vi "register_data_from_termocuple.vi"(8 "error in (no error)":errorcluster, 11 "DAQ Voltage in":refnum<class "DAQ Voltage.lvclass">) -> (0 "error out":errorcluster, 3 "DAQ Voltage out":refnum<class "DAQ Voltage.lvclass">)   [LabVIEW 2025, in "DAQ Voltage.lvlib" / "DAQ Voltage.lvclass"]
uses:
  DAQ Voltage.lvclass
  DAQ Voltage.lvclass/DAQ Voltage.ctl
  <vilib>/numeric/Random Number (Range) DBL.vi
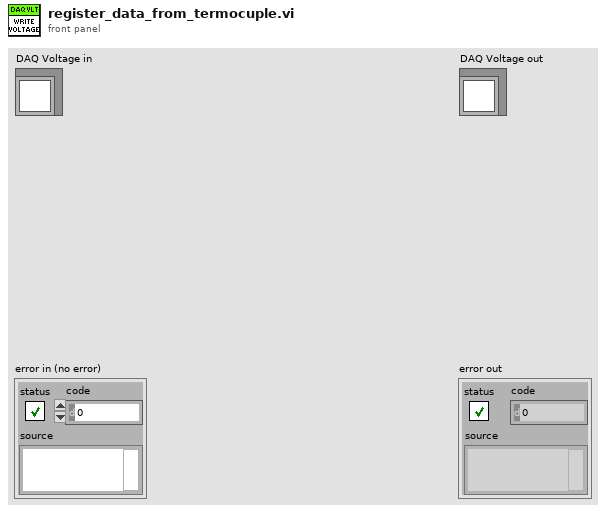
[diagram p1: front panel]
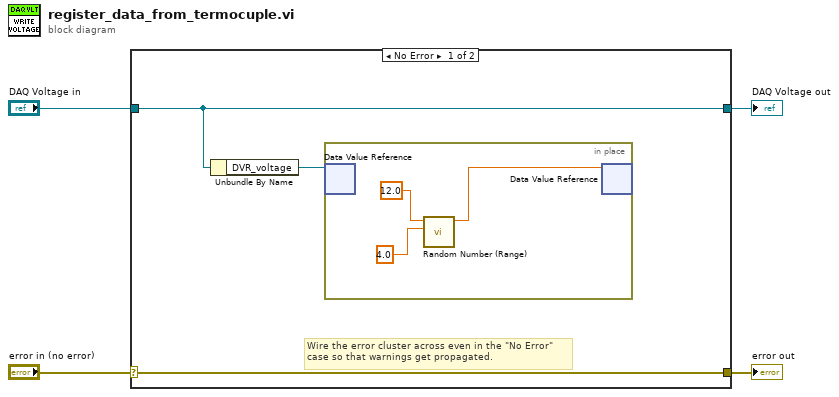
[diagram p0: block diagram]
diagram:
  n1 = case shown="No Error" "error in (no error)" {
    selector: "error in (no error)" -> [w7 w12]
    tunnel: [w7 w12] -> w3
    tunnel: [w6 w11] -> w1
    tunnel: "DAQ Voltage in" -> [w6 w11]
    frame No Error {
      # "Wire the error cluster across even in the \"No Error\"\ncase so that warnings get propagated."
      n2 = Unbundle By Name(w6) -> ("DVR_voltage"=w5:refnum<data-value>)
      n3 = in-place {
        n4 = in-place-dvr #1(w5) -> ()  [unwired: 2 out]
        n5 = call-poly <vilib>:"Random Number (Range).vi"("lower bound (0)"=4.0, "upper bound (100)"=12.0) -> ("number"=w8:dbl)  [unwired: 9 in]
        n6 = in-place-dvr #1(w8) -> ()  [unwired: 2 out]
      }
    }
    frame Error {
    }
  }
  "error out" <- w3
  "DAQ Voltage out" <- w1
